vi "Increment Time (timespec).vi"(8 "error in (no error)":errorcluster, 10 "nanos offset":i64, 11 "timespec in":cluster{"sec":u64, "nsec":u64}) -> (0 "error out":errorcluster, 3 "timespec out":cluster{"sec":u64, "nsec":u64})   [LabVIEW 2013, in "Linux RT Utilities.lvlib"]
doc: "This VI increments the provided timespec by a number of nanoseconds."
uses:
  Linux RT Utilities.lvlib
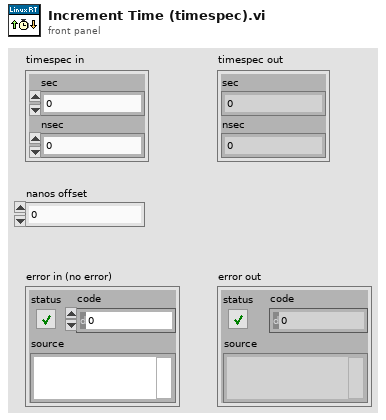
[diagram p1: front panel]
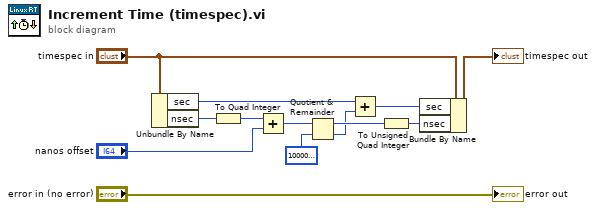
[diagram p0: block diagram]
diagram:
  n1 = Unbundle By Name("timespec in") -> ("sec"=w8:u64, "nsec"=w13:u64)
  n2 = To Quad Integer(1:w13) -> (0:w6:i64)
  n3 = Add(x=w6, y="nanos offset") -> (x+y=w4:i64)
  n4 = Quotient & Remainder(x=w4, y=i64 1000000000) -> (x-y*floor(x/y)=w3:i64, floor(x/y)=w1:i64)
  n5 = Add(x=w8, y=w1) -> (x+y=w10:u64)
  n6 = To Unsigned Quad Integer(1:w3) -> (0:w7:u64)
  n7 = Bundle By Name(cluster="timespec in", "sec"=w10, "nsec"=w7) -> (→"timespec out":cluster{"sec":u64, "nsec":u64})
  "error out" <- "error in (no error)"
